vi "Set_Argument.vi"(1 "Enable":bool, 2 "Argument":string, 3 "Argument List In":string[](array[string])) -> (0 "Argument List Out":string[](array[string]))   [LabVIEW 2011]
doc: "This VI sets the value of a boolean argument in the argument list. The value of a boolean argument is determined only by its existance as a string in the argument list array. For example, if the user wishes to set the argument \"SomeArgument\", it will be appended to the argument list if it is not already present. Conversely, if the user wishes to unset the argument \"SomeArgument\", that value will be deleted from the argument list, if it is present."
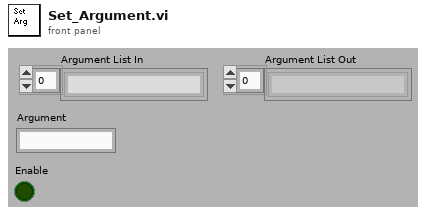
[diagram p1: front panel]
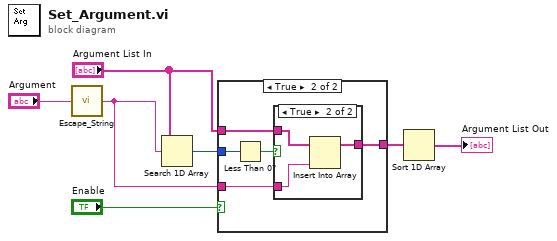
[diagram p0: block diagram]
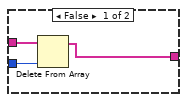
[diagram p2: hidden frame]
diagram:
  n1 = call "Escape_String.vi"("Input String"="Argument") -> ("Escaped String"=w1:string)
  n2 = Search 1D Array(1D array="Argument List In", element=w1) -> (index of element=w7:i32)  [unwired: 1 out]
  n3 = case shown="True" "Enable" {
    tunnel: "Argument List In" -> [w10 w13]
    tunnel: w7 -> [w9 w14]
    tunnel: w1 -> [_ w12]
    tunnel: [w8 w11] -> w6
    frame False {
      n4 = Delete From Array(array=w10, index=w9) -> (array with subset deleted=w8:string[])  [unwired: 1 in, 1 out]
    }
    frame True {
      n5 = Less Than 0?(x=w14) -> (x < 0?=w15:bool)
      n6 = case shown="True" w15 {
        tunnel: w13 -> [w16 w19]
        tunnel: w12 -> [_ w18]
        tunnel: [w16 w17] -> w11
        frame False {
        }
        frame True {
          n7 = Insert Into Array(array=w19, new element=w18) -> (w17:string[])  [unwired: 1 in]
        }
      }
    }
  }
  n8 = Sort 1D Array(array=w6) -> (sorted array=→"Argument List Out":string[])
